vi "Keithley DMM7510 Digitize for Average Current.vi"() -> ()   [LabVIEW 2025]
uses:
  Keithley DMM7510.lvlib
panel:
  out "Waveform Graph":cluster{dbl, dbl, dbl[]}(graph)={0.0, 1e-05, []}
  out "Full Output Data Path":path
  out "Average Current":dbl
  out "Actual Readings":i32
  out "Measurements":dbl[](array[numeric])
  in  "Reading Extraction Size":i32=1000
  in  "Sample Rate":dbl=100000.0
  in  "Sample Count":i32=1000000 min=10 step=1
  in  "Buffer Name":string="myBuffer"
  out "error out":errorcluster
  in  "Manual Range":dbl=1.0
  in  "error in (no error)":errorcluster
  in  "Function":u16(ring)=1 items=["Digitize Voltage", "Digitize Current"]
  in  "VISA resource name":refnum<visa-resource-name>
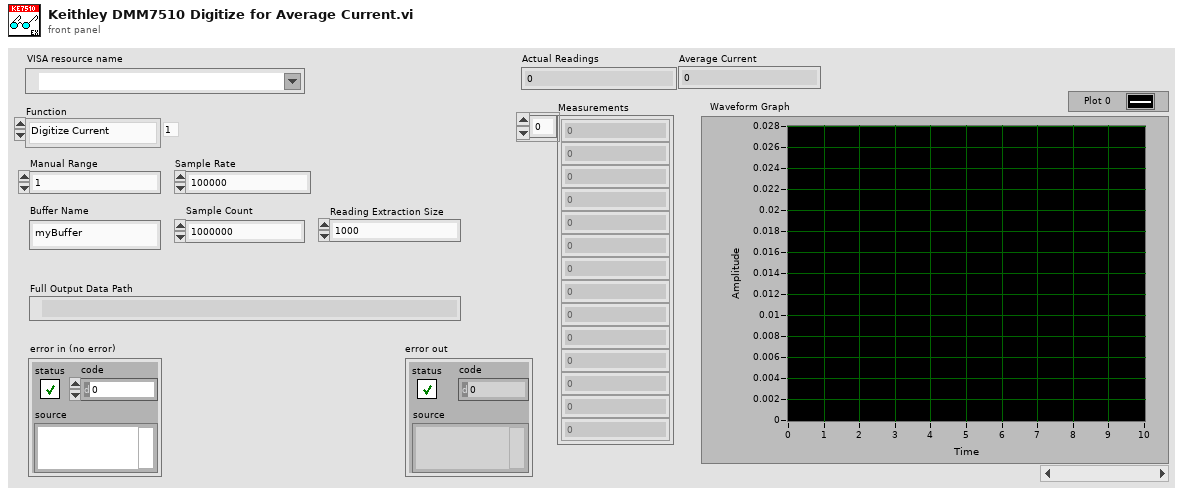
[diagram p1: front panel]
types:
  T1 = enum16{"In", "Out", "Open Drain", "Acceptor", "Master"}
  T2 = enum16{"open", "replace", "create", "open or create", "replace or create", "replace or create with confirmation"}
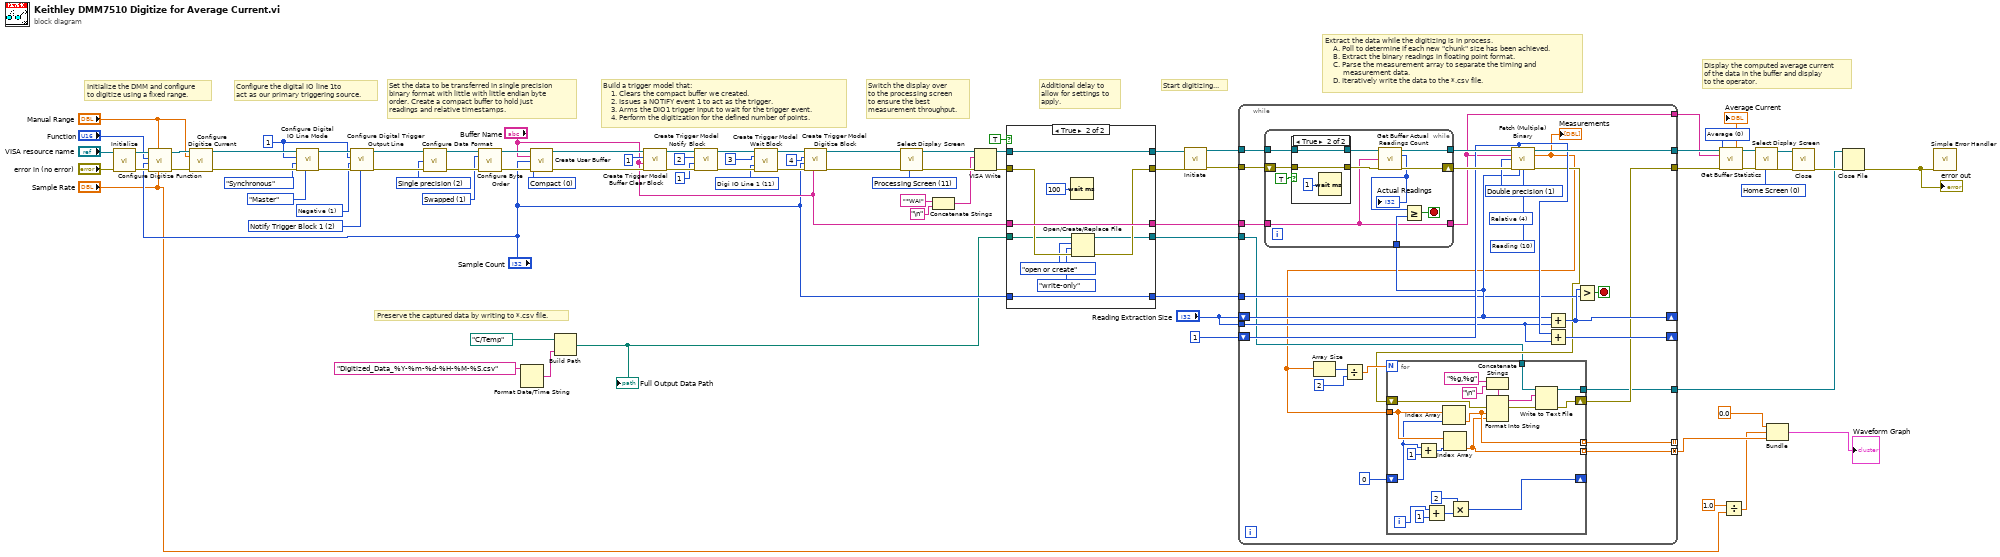
[diagram p0: block diagram]
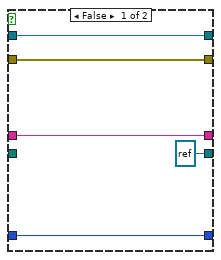
[diagram p3: hidden frame]
diagram:
  w8 = 0 items=["Average", "Maximum", "Minimum", "Peak-to-peak", "Standard deviation"] ("Statistics Type")
  w33 = u16 0 items=["Home Screen", "Home Large Reading", "Reading Sheet", "Graph Screen", "Histogram", "Functions Swipe", "Graph Swipe", "Secondary Swipe", "Settings Swipe", "Statistics Swipe", "User Swipe", "Processing Screen"] ("Screen Home")
  w44 = u16 11 items=["Home Screen", "Home Large Reading", "Reading Sheet", "Graph Screen", "Histogram", "Functions Swipe", "Graph Swipe", "Secondary Swipe", "Settings Swipe", "Statistics Swipe", "User Swipe", "Processing Screen"] ("Screen Home")
  w47 = u16 11 items=["None", "Front Pannel Trigger Key", "Notify Trigger Block 1", "Notify Trigger Block 2", "Notify Trigger Block 3", "Notify Trigger Block 4", "Notify Trigger Block 5", "Notify Trigger Block 6", "Notify Trigger Block 7", "Notify Trigger Block 8", "Command", "Digi IO Line 1", "Digi IO Line 2", "Digi IO Line 3", "Digi IO Line 4", "Digi IO Line 5", "Digi IO Line 6", "TSP-Link 1", "TSP-Link 2", "TSP-Link 3", "LAN 1", "LAN 2", "LAN 3", "LAN 4", "LAN 5", "LAN 6", "LAN 7", "LAN 8", "Blender 1", "Blender 2", "Timer 1", "Timer 2", "Timer 3", "Timer 4", "Analog Trigger", "External Trigger"] ("Event")
  w61 = 0 items=["Compact", "Standard", "Full", "Writable", "Full Writable"] ("Buffer Style (1: Standard)")
  w64 = u16 1 items=["Normal", "Swapped"] ("Byte Order")
  w65 = u16 2 items=["ASCII", "Double precision", "Single precision"] ("Byte Order")
  w70 = u16 2 items=["None", "Front Pannel Trigger Key", "Notify Trigger Block 1", "Notify Trigger Block 2", "Notify Trigger Block 3", "Notify Trigger Block 4", "Notify Trigger Block 5", "Notify Trigger Block 6", "Notify Trigger Block 7", "Notify Trigger Block 8", "Command", "Digi IO Line 1", "Digi IO Line 2", "Digi IO Line 3", "Digi IO Line 4", "Digi IO Line 5", "Digi IO Line 6", "TSP-Link 1", "TSP-Link 2", "TSP-Link 3", "LAN 1", "LAN 2", "LAN 3", "LAN 4", "LAN 5", "LAN 6", "LAN 7", "LAN 8", "Blender 1", "Blender 2", "Timer 1", "Timer 2", "Timer 3", "Timer 4", "Analog Trigger", "External Trigger"] ("Stimulus Event")
  w71 = u16 1 items=["Positive", "Negative"] ("Trigger Logic Type")
  w74 = u32 1 ("Digital IO Line (1)")
  # "Display the computed average current\nof the data in the buffer and display \nto the operator."
  # "Extract the data while the digitizing is in process.\n    A. Poll to determine if each new \"chunk\" size has been achieved.\n    B. Extract the binary readings in floating point format.\n    C. Parse the measurement array to separate the timing and\n         measurement data.\n    D. Iteratively write the data to the *.csv file."
  # "Preserve the captured data by writing to *.csv file."
  # "Start digitizing..."
  # "Additional delay to\nallow for settings to \napply."
  # "Switch the display over\nto the processing screen\nto ensure the best\nmeasurement throughput."
  # "Build a trigger model that:\n    1. Clears the compact buffer we created.\n    2. Issues a NOTIFY event 1 to act as the trigger.\n    3. Arms the DIO1 trigger input to wait for the trigger event. \n    4. Perform the digitization for the defined number of points."
  # "Set the data to be transferred in single precision \nbinary format with little with little endian byte \norder. Create a compact buffer to hold just \nreadings and relative timestamps."
  # "Configure the digital IO line 1to \nact as our primary triggering source."
  # "Initialize the DMM and configure\nto digitize using a fixed range."
  n1 = call "Initialize.vi"("error in (no error)"="error in (no error)", "VISA resource name"="VISA resource name") -> ("error out"=w83:errorcluster, "VISA resource name out"=w84:refnum<visa-resource-name>)  [unwired: 8 in]
  n2 = call "Configure Digitize Function.vi"("Sample Rate (1E+6)"="Sample Rate", "Manual Range (0)"="Manual Range", "error in (no error)"=w83, "Count (1)"="Sample Count", "Function"="Function", "VISA resource name"=w84) -> ("error out"=w81:errorcluster, "VISA resource name out"=w82:refnum<visa-resource-name>)  [unwired: 4 in]
  n3 = call "Configure Digitize Current.vi"("VISA resource name"=w82, "Manual Range"="Manual Range", "error in (no error)"=w81) -> ("VISA resource name out"=w78:refnum<visa-resource-name>, "error out"=w77:errorcluster)  [unwired: 11 in]
  n4 = call "Configure Digital IO Line Mode.vi"("Digital IO Mode (0: In)"=T1."Master", "error in (no error)"=w77, "Digital IO Trigger Type (0: Digital)"=enum16{"Digital", "Trigger", "Synchronous"}."Synchronous", "Digital IO Line (1)"=w74, "VISA resource name"=w78) -> ("error out"=w75:errorcluster, "VISA resource name out"=w76:refnum<visa-resource-name>)  [unwired: 5 in]
  n5 = call "Configure Digital Trigger Output Line.vi"("Stimulus Event"=w70, "error in (no error)"=w75, "Trigger Logic Type"=w71, "Digital IO Line (1)"=w74, "VISA resource name"=w76) -> ("error out"=w66:errorcluster, "VISA resource name out"=w67:refnum<visa-resource-name>)  [unwired: 5 in]
  n6 = call "Configure Data Format.vi"("VISA resource name"=w67, "Byte Order"=w65, "error in (no error)"=w66) -> ("VISA resource name out"=w69:refnum<visa-resource-name>, "error Out (no error)"=w68:errorcluster)  [unwired: 11 in]
  n7 = call "Configure Byte Order.vi"("VISA resource name"=w69, "Byte Order"=w64, "error in (no error)"=w68) -> ("VISA resource name out"=w63:refnum<visa-resource-name>, "error Out (no error)"=w62:errorcluster)  [unwired: 11 in]
  n8 = Format Date/Time String(time format string (%c)="Digitized_Data_%Y-%m-%d-%H-%M-%S.csv") -> (date/time string=w19:string)  [unwired: 2 in]
  n9 = call "Create User Buffer.vi"("VISA resource name"=w63, "Buffer Name"="Buffer Name", "Buffer Size"="Sample Count", "Buffer Style (1: Standard)"=w61, "error in (no error)"=w62) -> ("VISA resource name out"=w60:refnum<visa-resource-name>, "error out"=w59:errorcluster)  [unwired: 9 in]
  n10 = Build Path(base path=path "C:/Temp", name or relative path=w19) -> (appended path=w18:path)
  "Full Output Data Path" <- w18
  n11 = call "Create Trigger Model Buffer Clear Block.vi"("error in (no error)"=w59, "Buffer Name (defbuffer1)"="Buffer Name", "Block Number (1)"=1, "VISA resource name"=w60) -> ("error out"=w57:errorcluster, "VISA resource name out"=w58:refnum<visa-resource-name>)  [unwired: 6 in]
  n12 = call "Create Trigger Model Notify Block.vi"("error in (no error)"=w57, "Notify ID"=1, "Block Number (1)"=2, "VISA resource name"=w58) -> ("error out"=w56:errorcluster, "VISA resource name out"=w54:refnum<visa-resource-name>)  [unwired: 6 in]
  n13 = call "Create Trigger Model Wait Block.vi"("VISA resource name"=w54, "Block Number (1)"=3, "Event"=w47, "error in (no error)"=w56) -> ("VISA resource name out"=w53:refnum<visa-resource-name>, "error Out (no error)"=w55:errorcluster)  [unwired: 10 in]
  n14 = call "Create Trigger Model Digitize Block.vi"("Buffer Name (defbuffer1)"="Buffer Name", "error in (no error)"=w55, "Count"="Sample Count", "Block Number (1)"=4, "VISA resource name"=w53) -> ("error out"=w45:errorcluster, "VISA resource name out"=w46:refnum<visa-resource-name>)  [unwired: 5 in]
  n15 = call "Select Display Screen.vi"("error in (no error)"=w45, "Screen Home"=w44, "VISA resource name"=w46) -> ("error out"=w40:errorcluster, "VISA resource name out"=w41:refnum<visa-resource-name>)  [unwired: 7 in]
  n16 = Concatenate Strings("*WAI" ("string"), "\n") -> (w39:string)
  n17 = VISA Write(VISA resource name=w41, write buffer=w39, error in (no error)=w40) -> (VISA resource name out=w37:refnum<visa-resource-name>, error out=w36:errorcluster)  [unwired: 1 out]
  n18 = case shown="True" TRUE {
    tunnel: w37 -> [w90 w99]
    tunnel: w36 -> [w89 w96]
    tunnel: [w90 w99] -> w34
    tunnel: [w89 w95] -> w35
    tunnel: "Buffer Name" -> [w88 w98]
    tunnel: [w88 w98] -> w26
    tunnel: "Sample Count" -> [w87 w97]
    tunnel: [w87 w97] -> w22
    tunnel: w18 -> [_ w94]
    tunnel: [refnum<file> refnum ("refnum out") w91] -> w17
    frame False {
    }
    frame True {
      n19 = Wait (ms)(milliseconds to wait=u32 100) -> ()  [unwired: 1 out]
      n20 = Open/Create/Replace File(file path (use dialog)=w94, error in=w96, operation (0:open)=T2."open or create", access (0:read/write)=enum16{"read/write", "read-only", "write-only"}."write-only") -> (refnum out=w91:refnum<file>, error out=w95:errorcluster)  [unwired: 2 in, 1 out]
    }
  }
  n21 = call "Initiate.vi"("error in (no error)"=w35, "VISA resource name"=w34) -> ("error out"=w28:errorcluster, "VISA resource name out"=w29:refnum<visa-resource-name>)  [unwired: 8 in]
  n22 = while {
    tunnel: w29 -> [w128]
    tunnel: w28 -> [w127]
    tunnel: w26 -> [w126]
    tunnel: [w124] -> w11
    tunnel: [w108] -> w13
    shift-right: [w115] -> _
    shift-left: "Reading Extraction Size" -> [w118]
    shift-right: [w119] -> _
    shift-left: 1 ("Start Index (1)") -> [w120]
    tunnel: "Reading Extraction Size" -> [w117]
    tunnel: w22 -> [w114]
    tunnel: w17 -> [w107]
    tunnel: [w106] -> w14
    tunnel: [w104] -> w9
    tunnel: [w102] -> _ mode=indexing
    tunnel: [w101] -> w5 mode=concatenating
    stop <- w116 stop-if-true
    w105 = u16 10 items=["Date", "Extra", "Formatted", "Fractional", "Relative", "Seconds", "Status", "Time", "Timestamp", "Unit", "Reading"] ("Buffer Elements  2")
    w121 = u16 4 items=["Date", "Extra", "Formatted", "Fractional", "Relative", "Seconds", "Status", "Time", "Timestamp", "Unit"] ("Buffer Elements 1")
    w122 = u16 1 items=["Single precision", "Double precision"] ("Data Format")
    n23 = while {
      tunnel: w128 -> [w159]
      tunnel: [w155] -> w125
      shift-right: [w154] -> w123
      shift-left: w127 -> [w158]
      tunnel: w126 -> [w149]
      tunnel: w118 -> [w150]
      tunnel: [w149] -> w104
      stop <- w152 stop-if-true
      n24 = case shown="True" TRUE {
        tunnel: w159 -> [w161 w164]
        tunnel: [w161 w164] -> w157
        tunnel: w158 -> [w160 w163]
        tunnel: [w160 w163] -> w156
        frame False {
        }
        frame True {
          n25 = Wait (ms)(milliseconds to wait=u32 1) -> ()  [unwired: 1 out]
        }
      }
      n26 = call "Get Buffer Actual Readings Count.vi"("VISA resource name"=w157, "Buffer Name (defbuffer1)"=w149, "error in (no error)"=w156) -> ("VISA resource name out"=w155:refnum<visa-resource-name>, "Actual Readings"=w151:i32, "error out"=w154:errorcluster)  [unwired: 10 in]
      "Actual Readings" <- w151
      n27 = Greater Or Equal?(x=w151, y=w150) -> (x >= y?=w152:bool)
    }
    n28 = call "Fetch (Multiple) Binary.vi"("VISA resource name"=w125, "Start Index (1)"=w120, "Buffer Elements 1"=w121, "Buffer Name ()"=w104, "Data Format"=w122, "error in (no error)"=w123, "End Index (10)"=w118, "Buffer Elements  2"=w105) -> ("VISA resource name out"=w124:refnum<visa-resource-name>, "Measurements"=w103:dbl[], "error out"=w109:errorcluster)  [unwired: 5 in]
    "Measurements" <- w103
    n29 = Array Size(array=w103) -> (size(s)=w113:i32)
    n30 = Divide(x=w113, y=2) -> (x/y=w111:dbl)
    n31 = for {
      N: w111 -> [_]
      tunnel: w103 -> [w148]
      shift-right: [w140] -> _
      shift-left: 0 ("index") -> [w146]
      shift-right: [w134] -> w108
      shift-left: w109 -> [w139]
      tunnel: w107 -> [w132]
      tunnel: [w131] -> w106
      tunnel: [w130] -> w102 mode=indexing
      tunnel: [w129] -> w101 mode=indexing
      i -> [w143]
      n32 = Add(x=w146, y=1) -> (x+y=w147:i32)
      n33 = Add(x=w143, y=1) -> (x+y=w142:i32)
      n34 = Index Array(array=w148, index=w146) -> (element=w130:dbl)
      n35 = Index Array(array=w148, index=w147) -> (element=w129:dbl)
      n36 = Multiply(x=2, y=w142) -> (x*y=w140:i32)
      n37 = Concatenate Strings("%g,%g" ("string"), "\n") -> (w138:string)
      n38 = Format Into String(format string=w138, error in=w139, w130, w129) -> (resulting string=w133:string, error out=w135:errorcluster)  [unwired: 1 in]
      n39 = Write to Text File(file (use dialog)=w132, text=w133, error in=w135) -> (refnum out=w131:refnum<file>, error out=w134:errorcluster)  [unwired: 1 in, 1 out]
    }
    n40 = Add(x=w118, y=w117) -> (x+y=w115:i32)
    n41 = Add(x=w120, y=w117) -> (x+y=w119:i32)
    n42 = Greater?(x=w115, y=w114) -> (0:w116:bool)
  }
  n43 = call "Get Buffer Statistics.vi"("VISA resource name"=w11, "Buffer Name (defbuffer1)"=w9, "Statistics Type"=w8, "error in (no error)"=w13) -> ("VISA resource name out"=w10:refnum<visa-resource-name>, "Statistics Value"=→"Average Current":dbl, "error out"=w12:errorcluster)  [unwired: 9 in]
  n44 = Divide(x=1.0, y="Sample Rate") -> (x/y=w2:dbl)
  n45 = call "Select Display Screen.vi"("error in (no error)"=w12, "Screen Home"=w33, "VISA resource name"=w10) -> ("error out"=w31:errorcluster, "VISA resource name out"=w32:refnum<visa-resource-name>)  [unwired: 7 in]
  n46 = Bundle(0.0, w2, w5) -> (→"Waveform Graph":cluster{dbl, dbl, dbl[]})  [unwired: 1 in]
  n47 = call "Close.vi"("error in (no error)"=w31, "VISA resource name"=w32) -> ("error out"=w16:errorcluster)  [unwired: 9 in]
  n48 = Close File(refnum=w14, error in=w16) -> (error out=w15:errorcluster)  [unwired: 1 out]
  "error out" <- w15
  n49 = call <vilib>:"Simple Error Handler.vi"("error in (no error)"=w15) -> ()  [unwired: 4 in, 5 out]
